vi "GV line sync.vi"() -> ()   [LabVIEW 2017]
panel:
  out "Line sync":bool
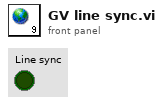
[diagram p1: front panel]
diagram:
